vi "Stopwatch, Popup.vi"(7 "Stop (Bool) Refnum":refnum<vi>, 8 "error in (no error)":errorcluster, 10 "Time Target":dbl[unit]=1.0 caption="Time Target (s)", 11 "Front Panel Window:Title":string="Waiting for File") -> (0 "error out":errorcluster {"code" format="%.0x"}, 2 "Time has Elapsed":bool, 3 "Elapsed Time (Knob)":dbl[unit](knob) scale=0.0..10.0)   [LabVIEW 2020]
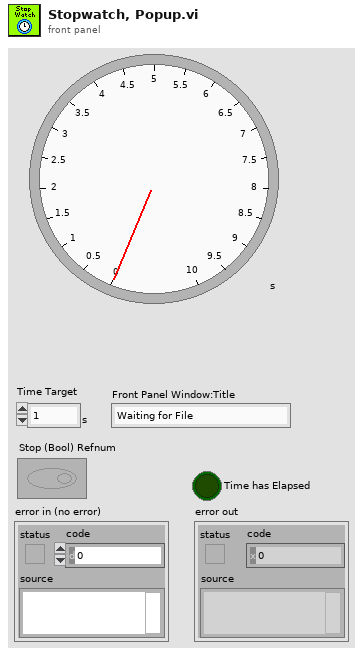
[diagram p1: front panel]
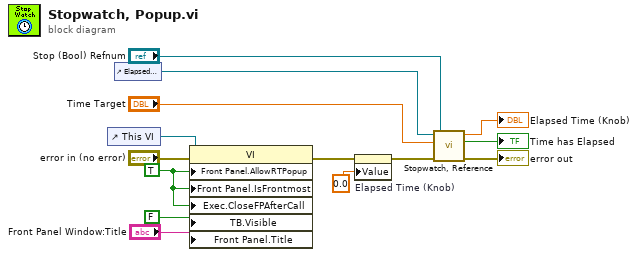
[diagram p0: block diagram]
diagram:
  w10 = TRUE ("Front Panel Window:Allow Runtime PopUp")
  n1 = control-ref of="This VI"() -> (w14:refnum<vi>)
  n2 = control-ref of="Elapsed Time (Knob)"() -> (w6:refnum<vi>)
  n3 = property class="VI"(reference=w14, error in="error in (no error)", "Front Panel.AllowRTPopup"=w10, "Front Panel.IsFrontmost"=w10, "Exec.CloseFPAfterCall"=w10, "TB.Visible"=FALSE ("Front Panel Window:Allow Runtime PopUp"), "Front Panel.Title"="Front Panel Window:Title") -> (error out=w3:errorcluster)  [unwired: 1 out]
  n4 = property on="Elapsed Time (Knob)" class="Knob (strict)"(error in=w3, "Value"=dbl[unit] 0.0 ("Elapsed Time (Knob)")) -> (error out=w2:errorcluster)  [unwired: 1 in, 1 out]
  n5 = call "Stopwatch, Reference.vi"("Stop (Bool) Refnum"="Stop (Bool) Refnum", "error in"=w2, "Time Target (10s)"="Time Target", "Stopwatch (Knob) Refnum"=w6) -> ("error out"=→"error out":errorcluster, "Time has Elapsed"=→"Time has Elapsed":bool, "Elapsed Time"=→"Elapsed Time (Knob)":dbl[unit])  [unwired: 5 in]
